vi "Init (subVi).vi"(0 "config file":path=path "C:/Users/guigue/Documents/hardware/software_config/rga/RGAConfig.ini") -> (1 "queue out":refnum<queue>, 2 "error (out)":errorcluster)   [LabVIEW 2016]
uses:
  global/Config_Infos.vi
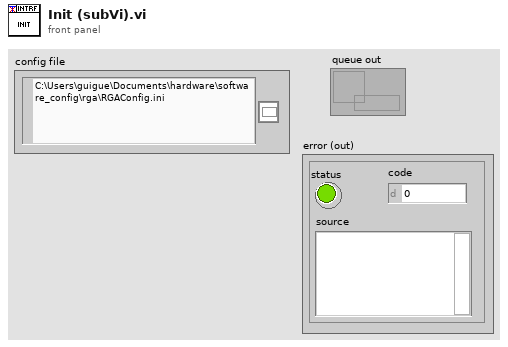
[diagram p1: front panel]
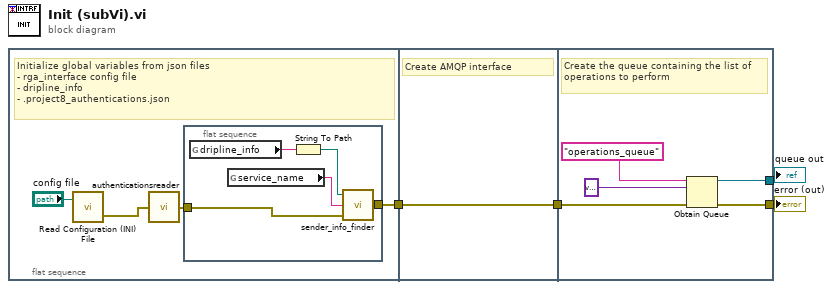
[diagram p0: block diagram]
diagram:
  n1 = flat-sequence {
    tunnel: [w6] -> w2
    tunnel: w2 -> [w14]
    tunnel: [w14] -> w1
    tunnel: [w15] -> w4
    tunnel: w1 -> [w16]
    tunnel: [w17] -> w3
    frame #0 {
      # "Initialize global variables from json files\n- rga_interface config file\n- dripline_info\n- .project8_authentications.json"
      n2 = call "Read Configuration (INI) File.vi"("configuration file path"="config file") -> ("error out"=w8:errorcluster)  [unwired: 2 in]
      n3 = call "authenticationsreader.vi"("error (in)"=w8) -> ("error (out)"=w7:errorcluster)
      n4 = flat-sequence {
        tunnel: w7 -> [w13]
        tunnel: [w12] -> w6
        frame #0 {
          n5 = global read "Config_Infos.vi" "dripline_info"() -> (w11:string)
          n6 = global read "Config_Infos.vi" "service_name"() -> (w9:string)
          n7 = String To Path(string=w11) -> (path=w10:path)
          n8 = call "sender_info_finder.vi"("error (in)"=w13, "service name"=w9, "file (use dialog)"=w10) -> ("error (out)"=w12:errorcluster)
        }
      }
    }
    frame #1 {
      # "Create AMQP interface"
    }
    frame #2 {
      # "Create the queue containing the list of operations to perform"
      n9 = Obtain Queue(name (unnamed)="operations_queue", element data type=variant, error in (no error)=w16) -> (queue out=w17:refnum<queue>, error out=w15:errorcluster)  [unwired: 2 in, 1 out]
    }
  }
  "error (out)" <- w4
  "queue out" <- w3
